vi "Ben LVComm.vi"() -> ()   [LabVIEW 2013]
panel:
  out "2D Picture":picture
  in  "Send Button":bool
  in  "GAIN2":dbl
  in  "GAIN1":dbl
  out "Rec Extra 4 Angle":dbl=255.0
  out "Rec Extra 3 Velocity":dbl=255.0
  out "Y":dbl=0.5
  out "X":dbl=0.5
  in  "Size of Rectangle":dbl=25.0
  in  "Display History":bool=TRUE
  in  "stop":bool
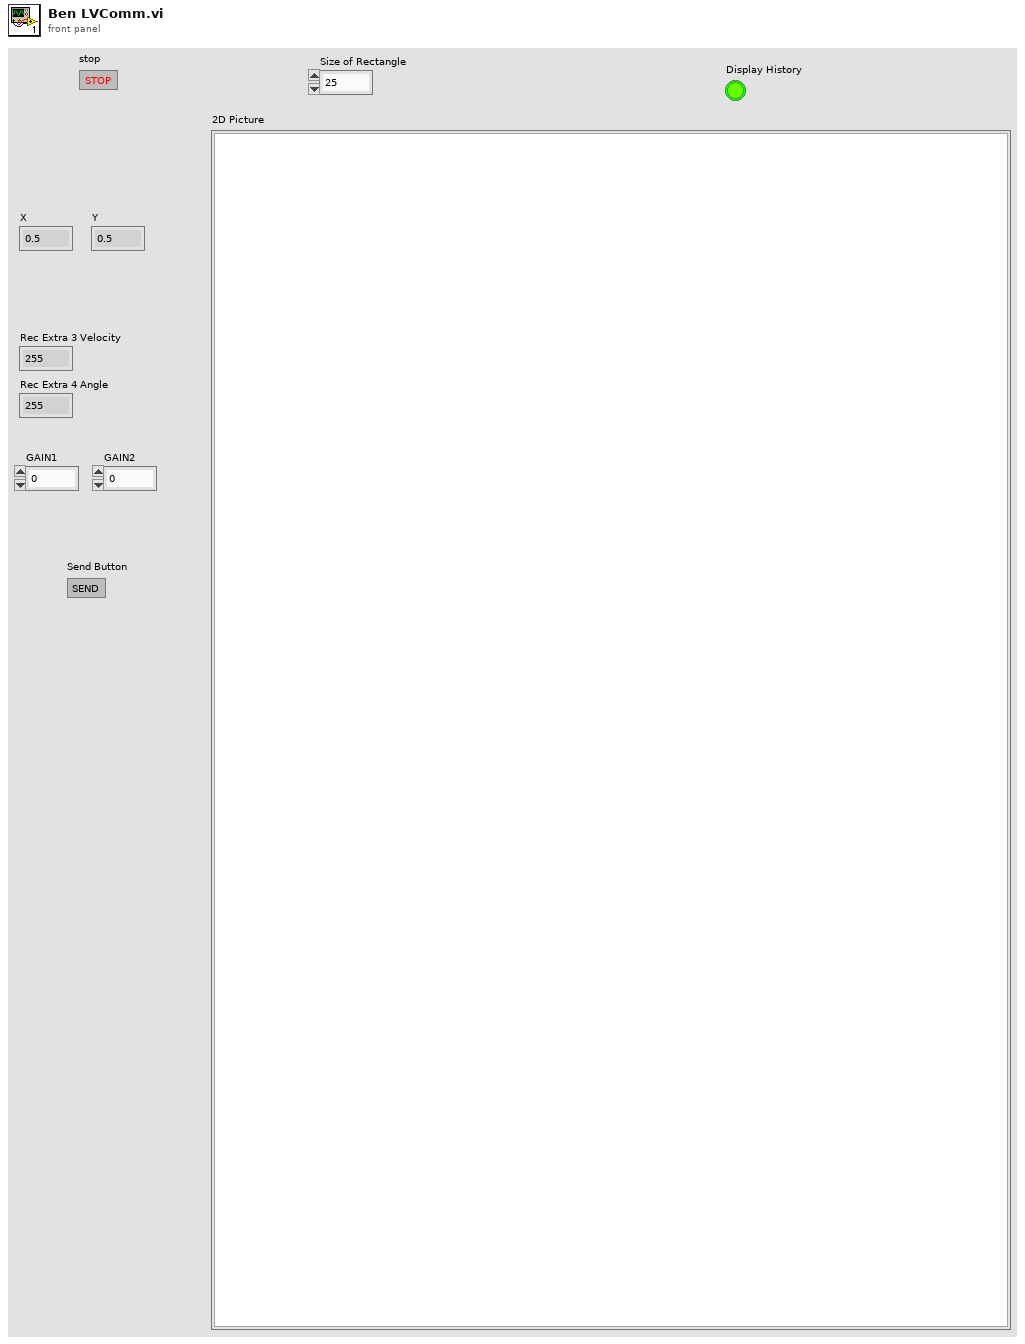
[diagram p1: front panel]
types:
  T1 = cluster{"Width":u16, "Style":enum32{"Solid", "Dash", "Dot", "DashDot", "DashDotDot"}}
  T2 = enum16{"Standard", "Buffered", "CRLF", "Immediate"}
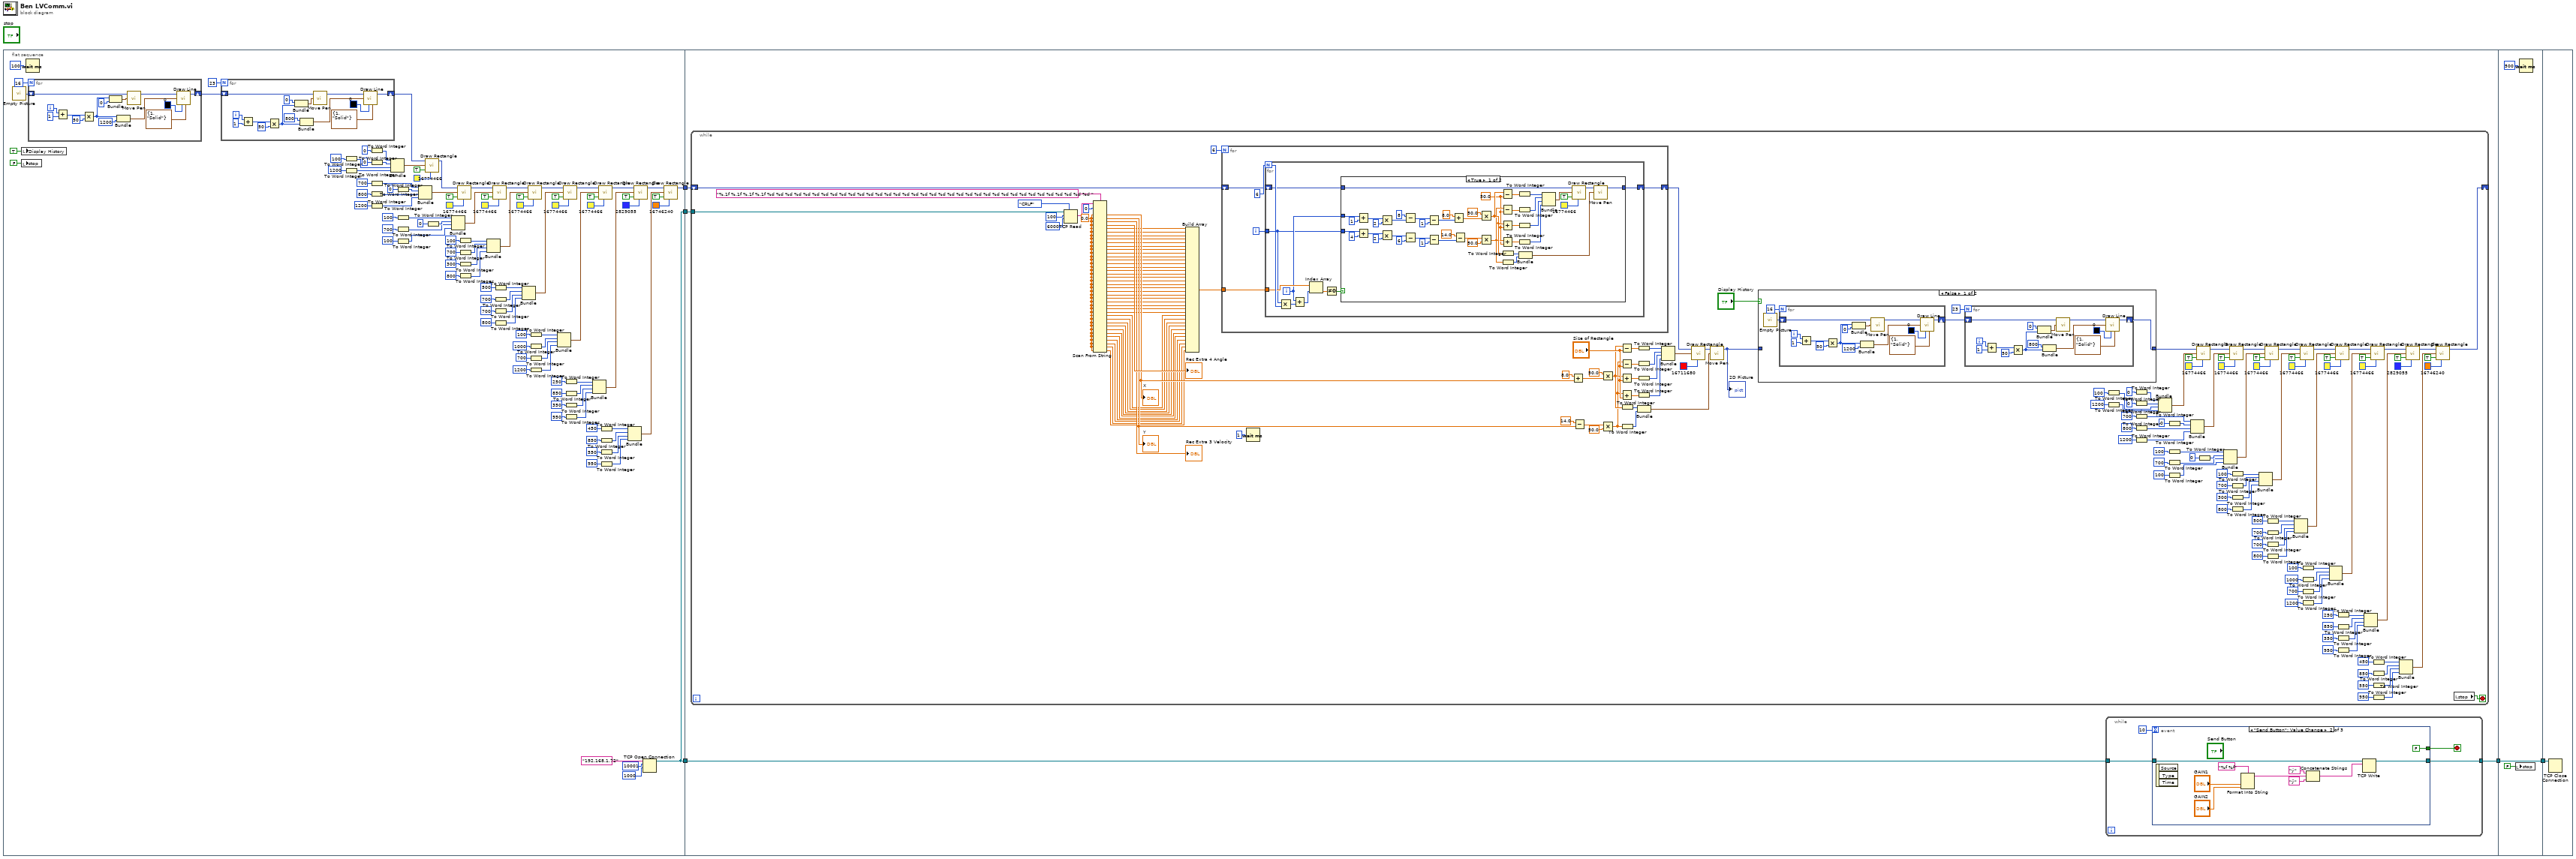
[diagram p0: block diagram]
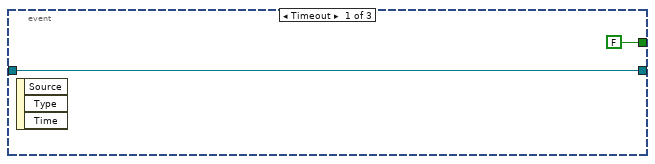
[diagram p4: hidden frame]
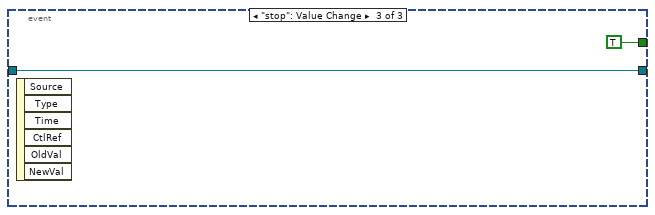
[diagram p5: hidden frame]
diagram:
  n1 = flat-sequence {
    tunnel: [w6] -> w5
    tunnel: [w107] -> w4
    tunnel: [w107] -> w3
    tunnel: w5 -> [w145]
    tunnel: w4 -> [w144]
    tunnel: w3 -> [w143]
    tunnel: [w142] -> w1
    tunnel: [w434] -> w2
    tunnel: w1 -> [w434]
    tunnel: w2 -> [w437]
    frame #0 {
      n2 = call "Empty Picture"() -> ("empty picture"=w106:picture)
      n3 = local write "Display History"(TRUE) -> ()
      n4 = local write "stop"(FALSE) -> ()
      n5 = Wait (ms)(milliseconds to wait=u32 100) -> ()  [unwired: 1 out]
      n6 = for {
        N: 16 -> [_]
        shift-right: [w130] -> w104
        shift-left: w106 -> [w141]
        i -> [w137]
        n7 = Add(x=w137, y=1) -> (x+y=w139:i32)
        n8 = Multiply(x=w139, y=50) -> (x*y=w133:i32)
        n9 = Bundle(w133, 0) -> (w135:cluster{i32, i32})  [unwired: 1 in]
        n10 = Bundle(w133, 1200) -> (w131:cluster{i32, i32})  [unwired: 1 in]
        n11 = call <vilib>:"Move Pen.vi"("new position"=w135, "picture"=w141) -> ("new picture"=w134:picture)  [unwired: 3 in]
        n12 = call <vilib>:"Draw Line.vi"("picture"=w134, "end point"=w131, "color(black)"=u32 0, "pen"=T1 {"Width"=1, "Style"=enum."Solid"}) -> ("new picture"=w130:picture)  [unwired: 5 in]
      }
      n13 = for {
        N: 23 -> [_]
        shift-right: [w119] -> w91
        shift-left: w104 -> [w127]
        i -> [w123]
        n14 = Add(x=w123, y=1) -> (x+y=w125:i32)
        n15 = Multiply(x=w125, y=50) -> (x*y=w114:i32)
        n16 = Bundle(0, w114) -> (w122:cluster{i32, i32})  [unwired: 1 in]
        n17 = Bundle(800, w114) -> (w120:cluster{i32, i32})  [unwired: 1 in]
        n18 = call <vilib>:"Move Pen.vi"("new position"=w122, "picture"=w127) -> ("new picture"=w121:picture)  [unwired: 3 in]
        n19 = call <vilib>:"Draw Line.vi"("picture"=w121, "end point"=w120, "color(black)"=u32 0, "pen"=T1 {"Width"=1, "Style"=enum."Solid"}) -> ("new picture"=w119:picture)  [unwired: 5 in]
      }
      n20 = To Word Integer(number=i16 100) -> (16bit integer=w100:i16)
      n21 = To Word Integer(number=i16 1200) -> (16bit integer=w99:i16)
      n22 = To Word Integer(number=0) -> (16bit integer=w102:i16)
      n23 = To Word Integer(number=i16 0) -> (16bit integer=w101:i16)
      n24 = To Word Integer(number=700) -> (16bit integer=w90:i16)
      n25 = To Word Integer(number=i16 800) -> (16bit integer=w88:i16)
      n26 = To Word Integer(number=i16 1200) -> (16bit integer=w87:i16)
      n27 = Bundle(w102, w101, w100, w99) -> (w98:cluster{i16, i16, i16, i16})  [unwired: 1 in]
      n28 = To Word Integer(number=i16 0) -> (16bit integer=w89:i16)
      n29 = To Word Integer(number=100) -> (16bit integer=w79:i16)
      n30 = To Word Integer(number=i16 700) -> (16bit integer=w77:i16)
      n31 = To Word Integer(number=i16 100) -> (16bit integer=w76:i16)
      n32 = Bundle(w90, w89, w88, w87) -> (w86:cluster{i16, i16, i16, i16})  [unwired: 1 in]
      n33 = call <vilib>:"Draw Rectangle.vi"("picture"=w91, "rect"=w98, "fill?(F)"=TRUE, "color(black)"=u32 16774466) -> ("new picture"=w35:picture)  [unwired: 5 in]
      n34 = To Word Integer(number=i16 0) -> (16bit integer=w78:i16)
      n35 = Bundle(w79, w78, w77, w76) -> (w75:cluster{i16, i16, i16, i16})  [unwired: 1 in]
      n36 = call <vilib>:"Draw Rectangle.vi"("picture"=w35, "rect"=w86, "fill?(F)"=TRUE, "color(black)"=u32 16774466) -> ("new picture"=w34:picture)  [unwired: 5 in]
      n37 = To Word Integer(number=100) -> (16bit integer=w68:i16)
      n38 = To Word Integer(number=i16 700) -> (16bit integer=w67:i16)
      n39 = To Word Integer(number=i16 300) -> (16bit integer=w66:i16)
      n40 = To Word Integer(number=i16 800) -> (16bit integer=w65:i16)
      n41 = Bundle(w68, w67, w66, w65) -> (w64:cluster{i16, i16, i16, i16})  [unwired: 1 in]
      n42 = call <vilib>:"Draw Rectangle.vi"("picture"=w34, "rect"=w75, "fill?(F)"=TRUE, "color(black)"=u32 16774466) -> ("new picture"=w33:picture)  [unwired: 5 in]
      n43 = To Word Integer(number=500) -> (16bit integer=w57:i16)
      n44 = To Word Integer(number=i16 700) -> (16bit integer=w56:i16)
      n45 = To Word Integer(number=i16 700) -> (16bit integer=w55:i16)
      n46 = To Word Integer(number=i16 800) -> (16bit integer=w54:i16)
      n47 = Bundle(w57, w56, w55, w54) -> (w53:cluster{i16, i16, i16, i16})  [unwired: 1 in]
      n48 = call <vilib>:"Draw Rectangle.vi"("picture"=w33, "rect"=w64, "fill?(F)"=TRUE, "color(black)"=u32 16774466) -> ("new picture"=w32:picture)  [unwired: 5 in]
      n49 = To Word Integer(number=100) -> (16bit integer=w46:i16)
      n50 = To Word Integer(number=i16 1000) -> (16bit integer=w45:i16)
      n51 = To Word Integer(number=i16 700) -> (16bit integer=w44:i16)
      n52 = To Word Integer(number=i16 1200) -> (16bit integer=w43:i16)
      n53 = Bundle(w46, w45, w44, w43) -> (w42:cluster{i16, i16, i16, i16})  [unwired: 1 in]
      n54 = call <vilib>:"Draw Rectangle.vi"("picture"=w32, "rect"=w53, "fill?(F)"=TRUE, "color(black)"=u32 16774466) -> ("new picture"=w31:picture)  [unwired: 5 in]
      n55 = To Word Integer(number=250) -> (16bit integer=w30:i16)
      n56 = To Word Integer(number=i16 850) -> (16bit integer=w29:i16)
      n57 = To Word Integer(number=i16 350) -> (16bit integer=w28:i16)
      n58 = To Word Integer(number=i16 950) -> (16bit integer=w27:i16)
      n59 = Bundle(w30, w29, w28, w27) -> (w26:cluster{i16, i16, i16, i16})  [unwired: 1 in]
      n60 = call <vilib>:"Draw Rectangle.vi"("picture"=w31, "rect"=w42, "fill?(F)"=TRUE, "color(black)"=u32 16774466) -> ("new picture"=w7:picture)  [unwired: 5 in]
      n61 = To Word Integer(number=450) -> (16bit integer=w19:i16)
      n62 = To Word Integer(number=i16 850) -> (16bit integer=w18:i16)
      n63 = To Word Integer(number=i16 550) -> (16bit integer=w17:i16)
      n64 = To Word Integer(number=i16 950) -> (16bit integer=w16:i16)
      n65 = Bundle(w19, w18, w17, w16) -> (w15:cluster{i16, i16, i16, i16})  [unwired: 1 in]
      n66 = call <vilib>:"Draw Rectangle.vi"("picture"=w7, "rect"=w26, "fill?(F)"=TRUE, "color(black)"=u32 2829055) -> ("new picture"=w8:picture)  [unwired: 5 in]
      n67 = TCP Open Connection(address="192.168.1.72", remote port or service name=u16 10001, timeout ms (60000)=1000) -> (connection ID=w107:refnum<k5>)  [unwired: 2 in, 1 out]
      n68 = call <vilib>:"Draw Rectangle.vi"("picture"=w8, "rect"=w15, "fill?(F)"=TRUE, "color(black)"=u32 16746240) -> ("new picture"=w6:picture)  [unwired: 5 in]
    }
    frame #1 {
      n69 = while {
        shift-right: [w147] -> _
        shift-left: w145 -> [w244]
        tunnel: w143 -> [w299]
        stop <- w300 stop-if-true
        w243 = 0.0 ("default value 1")
        n70 = TCP Read(connection ID=w299, bytes to read=100, 7:T2."CRLF" ("mode (standard)"), 9:6000 ("timeout ms (25000)")) -> (data out=w298:string)  [unwired: 1 in, 2 out]
        n71 = Scan From String(format string="%.1f %.1f %.1f %.1f %d %d %d %d %d %d %d %d %d %d %d %d %d %d %d %d %d %d %d %d %d %d %d %d %d %d %d %d %d %d %d %d %d %d %d %d ", input string=w298, initial scan location=u32 0, default 1=w243, default 2=w243, default 3=w243, default 4=w243, default 5=w243, default 6=w243, default 7=w243, default 8=w243, default 9=w243, default 10=w243, default 11=w243, default 12=w243, default 13=w243, default 14=w243, default 15=w243, default 16=w243, default 17=w243, default 18=w243, default 19=w243, default 20=w243, default 21=w243, default 22=w243, default 23=w243, default 24=w243, default 25=w243, default 26=w243, default 27=w243, default 28=w243, default 29=w243, default 30=w243, default 31=w243, default 32=w243, default 33=w243, default 34=w243, default 35=w243, default 36=w243, default 37=w243, default 38=w243, default 39=w243, default 40=w243) -> (output 1=w287:dbl, output 2=w285:dbl, output 3=→"Rec Extra 3 Velocity":dbl, output 4=→"Rec Extra 4 Angle":dbl, output 5=w283:dbl, output 6=w282:dbl, output 7=w281:dbl, output 8=w280:dbl, output 9=w279:dbl, output 10=w278:dbl, output 11=w277:dbl, output 12=w276:dbl, output 13=w275:dbl, output 14=w274:dbl, output 15=w273:dbl, output 16=w272:dbl, output 17=w271:dbl, output 18=w270:dbl, output 19=w269:dbl, output 20=w268:dbl, output 21=w267:dbl, output 22=w266:dbl, output 23=w265:dbl, output 24=w264:dbl, output 25=w263:dbl, output 26=w262:dbl, output 27=w261:dbl, output 28=w260:dbl, output 29=w259:dbl, output 30=w258:dbl, output 31=w257:dbl, output 32=w256:dbl, output 33=w255:dbl, output 34=w254:dbl, output 35=w253:dbl, output 36=w252:dbl, output 37=w251:dbl, output 38=w250:dbl, output 39=w249:dbl, output 40=w248:dbl)  [unwired: 1 in, 3 out]
        "X" <- w287
        "Y" <- w285
        n72 = Build Array(w283, w282, w281, w280, w279, w278, w277, w276, w275, w274, w273, w272, w271, w270, w269, w268, w267, w266, w265, w264, w263, w262, w261, w260, w259, w258, w257, w256, w255, w254, w253, w252, w251, w250, w249, w248) -> (w246:dbl[])
        n73 = for {
          N: 6 -> [_]
          tunnel: w246 -> [w324]
          shift-right: [w323] -> w245
          shift-left: w244 -> [w322]
          i -> [w325]
          n74 = for {
            N: 6 -> [w336]
            tunnel: w325 -> [w329]
            tunnel: w324 -> [w333]
            shift-right: [w328] -> w323
            shift-left: w322 -> [w327]
            i -> [w330]
            n75 = Multiply(x=w329, y=w336) -> (x*y=w335:i32)
            n76 = Add(x=w330, y=w335) -> (x+y=w334:i32)
            n77 = Index Array(array=w333, index=w334) -> (element=w332:dbl)
            n78 = Not Equal To 0?(x=w332) -> (x != 0?=w331:bool)
            n79 = case shown="True" w331 {
              tunnel: w327 -> [w346 w381]
              tunnel: w330 -> [w340 _]
              tunnel: w329 -> [w343 _]
              tunnel: [w344 w381] -> w328
              frame True {
                w350 = 50.0 ("y")
                n80 = Add(x=w340, y=1) -> (x+y=w339:i32)
                n81 = Add(x=w343, y=4) -> (x+y=w342:i32)
                n82 = Multiply(x=w339, y=2) -> (x*y=w379:i32)
                n83 = Multiply(x=w342, y=2) -> (x*y=w372:i32)
                n84 = Subtract(x=8, y=w379) -> (x-y=w377:i32)
                n85 = Subtract(x=w372, y=6) -> (x-y=w374:i32)
                n86 = Subtract(x=w377, y=1) -> (x-y=w349:i32)
                n87 = Subtract(x=w374, y=1) -> (x-y=w348:i32)
                n88 = Add(x=8.0, y=w349) -> (x+y=w356:dbl)
                n89 = Subtract(x=14.0, y=w348) -> (x-y=w351:dbl)
                n90 = Multiply(x=50.0, y=w356) -> (x*y=w355:dbl)
                n91 = Multiply(x=w351, y=50.0) -> (x*y=w354:dbl)
                n92 = Subtract(x=w355, y=w350) -> (x-y=w368:dbl)
                n93 = Subtract(x=w354, y=w350) -> (x-y=w367:dbl)
                n94 = Add(x=w355, y=w350) -> (x+y=w366:dbl)
                n95 = Add(x=w354, y=w350) -> (x+y=w365:dbl)
                n96 = To Word Integer(number=w355) -> (16bit integer=w358:i16)
                n97 = To Word Integer(number=w354) -> (16bit integer=w357:i16)
                n98 = To Word Integer(number=w368) -> (16bit integer=w364:i16)
                n99 = To Word Integer(number=w367) -> (16bit integer=w363:i16)
                n100 = To Word Integer(number=w366) -> (16bit integer=w362:i16)
                n101 = To Word Integer(number=w365) -> (16bit integer=w361:i16)
                n102 = Bundle(w358, w357) -> (w345:cluster{i16, i16})  [unwired: 1 in]
                n103 = Bundle(w364, w363, w362, w361) -> (w360:cluster{i16, i16, i16, i16})  [unwired: 1 in]
                n104 = call <vilib>:"Draw Rectangle.vi"("picture"=w346, "rect"=w360, "fill?(F)"=TRUE, "color(black)"=u32 16774466) -> ("new picture"=w347:picture)  [unwired: 5 in]
                n105 = call <vilib>:"Move Pen.vi"("new position"=w345, "picture"=w347) -> ("new picture"=w344:picture)  [unwired: 3 in]
              }
              frame False {
              }
            }
          }
        }
        n106 = Wait (ms)(milliseconds to wait=u32 1) -> ()  [unwired: 1 out]
        n107 = Add(x=8.0, y=w287) -> (x+y=w294:dbl)
        n108 = Subtract(x=14.0, y=w285) -> (x-y=w284:dbl)
        n109 = Multiply(x=50.0, y=w294) -> (x*y=w292:dbl)
        n110 = Multiply(x=w284, y=50.0) -> (x*y=w291:dbl)
        n111 = Subtract(x=w292, y="Size of Rectangle") -> (x-y=w311:dbl)
        n112 = Subtract(x=w291, y="Size of Rectangle") -> (x-y=w310:dbl)
        n113 = Add(x=w292, y="Size of Rectangle") -> (x+y=w309:dbl)
        n114 = Add(x=w291, y="Size of Rectangle") -> (x+y=w308:dbl)
        n115 = To Word Integer(number=w292) -> (16bit integer=w296:i16)
        n116 = To Word Integer(number=w291) -> (16bit integer=w295:i16)
        n117 = To Word Integer(number=w311) -> (16bit integer=w307:i16)
        n118 = To Word Integer(number=w310) -> (16bit integer=w306:i16)
        n119 = To Word Integer(number=w309) -> (16bit integer=w305:i16)
        n120 = To Word Integer(number=w308) -> (16bit integer=w304:i16)
        n121 = Bundle(w296, w295) -> (w297:cluster{i16, i16})  [unwired: 1 in]
        n122 = Bundle(w307, w306, w305, w304) -> (w303:cluster{i16, i16, i16, i16})  [unwired: 1 in]
        n123 = call <vilib>:"Draw Rectangle.vi"("picture"=w245, "rect"=w303, "color(black)"=u32 16711680) -> ("new picture"=w293:picture)  [unwired: 6 in]
        n124 = call <vilib>:"Move Pen.vi"("new position"=w297, "picture"=w293) -> ("new picture"=w289:picture)  [unwired: 3 in]
        "2D Picture" <- w289
        n125 = case shown="False" "Display History" {
          tunnel: [w383 w415] -> w171
          tunnel: w289 -> [_ w415]
          frame False {
            n126 = call "Empty Picture"() -> ("empty picture"=w386:picture)
            n127 = for {
              N: 16 -> [_]
              shift-right: [w403] -> w384
              shift-left: w386 -> [w414]
              i -> [w410]
              n128 = Add(x=w410, y=1) -> (x+y=w412:i32)
              n129 = Multiply(x=w412, y=50) -> (x*y=w406:i32)
              n130 = Bundle(w406, 0) -> (w408:cluster{i32, i32})  [unwired: 1 in]
              n131 = Bundle(w406, 1200) -> (w404:cluster{i32, i32})  [unwired: 1 in]
              n132 = call <vilib>:"Move Pen.vi"("new position"=w408, "picture"=w414) -> ("new picture"=w407:picture)  [unwired: 3 in]
              n133 = call <vilib>:"Draw Line.vi"("picture"=w407, "end point"=w404, "color(black)"=u32 0, "pen"=T1 {"Width"=1, "Style"=enum."Solid"}) -> ("new picture"=w403:picture)  [unwired: 5 in]
            }
            n134 = for {
              N: 23 -> [_]
              shift-right: [w392] -> w383
              shift-left: w384 -> [w400]
              i -> [w396]
              n135 = Add(x=w396, y=1) -> (x+y=w398:i32)
              n136 = Multiply(x=w398, y=50) -> (x*y=w387:i32)
              n137 = Bundle(0, w387) -> (w395:cluster{i32, i32})  [unwired: 1 in]
              n138 = Bundle(800, w387) -> (w393:cluster{i32, i32})  [unwired: 1 in]
              n139 = call <vilib>:"Move Pen.vi"("new position"=w395, "picture"=w400) -> ("new picture"=w394:picture)  [unwired: 3 in]
              n140 = call <vilib>:"Draw Line.vi"("picture"=w394, "end point"=w393, "color(black)"=u32 0, "pen"=T1 {"Width"=1, "Style"=enum."Solid"}) -> ("new picture"=w392:picture)  [unwired: 5 in]
            }
          }
          frame True {
          }
        }
        n141 = To Word Integer(number=i16 100) -> (16bit integer=w240:i16)
        n142 = To Word Integer(number=i16 1200) -> (16bit integer=w239:i16)
        n143 = To Word Integer(number=0) -> (16bit integer=w242:i16)
        n144 = To Word Integer(number=i16 0) -> (16bit integer=w241:i16)
        n145 = To Word Integer(number=700) -> (16bit integer=w231:i16)
        n146 = To Word Integer(number=i16 800) -> (16bit integer=w229:i16)
        n147 = To Word Integer(number=i16 1200) -> (16bit integer=w228:i16)
        n148 = Bundle(w242, w241, w240, w239) -> (w238:cluster{i16, i16, i16, i16})  [unwired: 1 in]
        n149 = To Word Integer(number=i16 0) -> (16bit integer=w230:i16)
        n150 = To Word Integer(number=100) -> (16bit integer=w220:i16)
        n151 = To Word Integer(number=i16 700) -> (16bit integer=w218:i16)
        n152 = To Word Integer(number=i16 100) -> (16bit integer=w217:i16)
        n153 = Bundle(w231, w230, w229, w228) -> (w227:cluster{i16, i16, i16, i16})  [unwired: 1 in]
        n154 = call <vilib>:"Draw Rectangle.vi"("picture"=w171, "rect"=w238, "fill?(F)"=TRUE, "color(black)"=u32 16774466) -> ("new picture"=w176:picture)  [unwired: 5 in]
        n155 = To Word Integer(number=i16 0) -> (16bit integer=w219:i16)
        n156 = Bundle(w220, w219, w218, w217) -> (w216:cluster{i16, i16, i16, i16})  [unwired: 1 in]
        n157 = call <vilib>:"Draw Rectangle.vi"("picture"=w176, "rect"=w227, "fill?(F)"=TRUE, "color(black)"=u32 16774466) -> ("new picture"=w175:picture)  [unwired: 5 in]
        n158 = To Word Integer(number=100) -> (16bit integer=w209:i16)
        n159 = To Word Integer(number=i16 700) -> (16bit integer=w208:i16)
        n160 = To Word Integer(number=i16 300) -> (16bit integer=w207:i16)
        n161 = To Word Integer(number=i16 800) -> (16bit integer=w206:i16)
        n162 = Bundle(w209, w208, w207, w206) -> (w205:cluster{i16, i16, i16, i16})  [unwired: 1 in]
        n163 = call <vilib>:"Draw Rectangle.vi"("picture"=w175, "rect"=w216, "fill?(F)"=TRUE, "color(black)"=u32 16774466) -> ("new picture"=w174:picture)  [unwired: 5 in]
        n164 = To Word Integer(number=500) -> (16bit integer=w198:i16)
        n165 = To Word Integer(number=i16 700) -> (16bit integer=w197:i16)
        n166 = To Word Integer(number=i16 700) -> (16bit integer=w196:i16)
        n167 = To Word Integer(number=i16 800) -> (16bit integer=w195:i16)
        n168 = Bundle(w198, w197, w196, w195) -> (w194:cluster{i16, i16, i16, i16})  [unwired: 1 in]
        n169 = call <vilib>:"Draw Rectangle.vi"("picture"=w174, "rect"=w205, "fill?(F)"=TRUE, "color(black)"=u32 16774466) -> ("new picture"=w173:picture)  [unwired: 5 in]
        n170 = To Word Integer(number=100) -> (16bit integer=w187:i16)
        n171 = To Word Integer(number=i16 1000) -> (16bit integer=w186:i16)
        n172 = To Word Integer(number=i16 700) -> (16bit integer=w185:i16)
        n173 = To Word Integer(number=i16 1200) -> (16bit integer=w184:i16)
        n174 = Bundle(w187, w186, w185, w184) -> (w183:cluster{i16, i16, i16, i16})  [unwired: 1 in]
        n175 = call <vilib>:"Draw Rectangle.vi"("picture"=w173, "rect"=w194, "fill?(F)"=TRUE, "color(black)"=u32 16774466) -> ("new picture"=w172:picture)  [unwired: 5 in]
        n176 = To Word Integer(number=250) -> (16bit integer=w170:i16)
        n177 = To Word Integer(number=i16 850) -> (16bit integer=w169:i16)
        n178 = To Word Integer(number=i16 350) -> (16bit integer=w168:i16)
        n179 = To Word Integer(number=i16 950) -> (16bit integer=w167:i16)
        n180 = Bundle(w170, w169, w168, w167) -> (w166:cluster{i16, i16, i16, i16})  [unwired: 1 in]
        n181 = call <vilib>:"Draw Rectangle.vi"("picture"=w172, "rect"=w183, "fill?(F)"=TRUE, "color(black)"=u32 16774466) -> ("new picture"=w146:picture)  [unwired: 5 in]
        n182 = To Word Integer(number=450) -> (16bit integer=w159:i16)
        n183 = To Word Integer(number=i16 850) -> (16bit integer=w158:i16)
        n184 = To Word Integer(number=i16 550) -> (16bit integer=w157:i16)
        n185 = To Word Integer(number=i16 950) -> (16bit integer=w156:i16)
        n186 = Bundle(w159, w158, w157, w156) -> (w155:cluster{i16, i16, i16, i16})  [unwired: 1 in]
        n187 = call <vilib>:"Draw Rectangle.vi"("picture"=w146, "rect"=w166, "fill?(F)"=TRUE, "color(black)"=u32 2829055) -> ("new picture"=w148:picture)  [unwired: 5 in]
        n188 = call <vilib>:"Draw Rectangle.vi"("picture"=w148, "rect"=w155, "fill?(F)"=TRUE, "color(black)"=u32 16746240) -> ("new picture"=w147:picture)  [unwired: 5 in]
        n189 = local read "stop"() -> (w300:bool)
      }
      n190 = while {
        tunnel: w144 -> [w418]
        tunnel: [w417] -> w142
        stop <- w416 stop-if-true
        n191 = event shown="[1] \"Send Button\": Value Change" {
          selector: _ -> [_ _ _]
          dyn-events: _ -> [_ _ _]
          timeout: 10 -> [_ _ _]
          tunnel: w418 -> [w421 w424 w432]
          tunnel: [w421 w423 w432] -> w417
          tunnel: [FALSE FALSE TRUE] -> w416
          event Timeout {
            n192 = event-data() -> ()  [unwired: 1 in, 3 out]
          }
          event "Send Button": Value Change {
            n193 = event-data() -> ()  [unwired: 1 in, 3 out]
            n194 = Format Into String(format string="%f %f", "GAIN1", "GAIN2") -> (resulting string=w426:string)  [unwired: 2 in, 1 out]
            n195 = Concatenate Strings("ý" ("string"), w426, "ÿ" ("string")) -> (w425:string)
            n196 = TCP Write(connection ID=w424, data in=w425) -> (connection ID out=w423:refnum<k5>)  [unwired: 2 in, 2 out]
          }
          event "stop": Value Change {
            n197 = event-data() -> ()  [unwired: 1 in, 6 out]
          }
        }
      }
    }
    frame #2 {
      n198 = local write "stop"(FALSE) -> ()
      n199 = Wait (ms)(milliseconds to wait=u32 500) -> ()  [unwired: 1 out]
    }
    frame #3 {
      n200 = TCP Close Connection(connection ID=w437) -> ()  [unwired: 2 in, 2 out]
    }
  }
